vi "PH_Beckhoff_StepMot.calc Activity.vi"(1 "Endswitch?":bool, 2 "Moving":bool, 3 "ADS Error in":i32, 4 "Status":T1) -> (0 "Axis Activity":T4)   [LabVIEW 2014, in "PH_Beckhoff_StepMot.lvlib"]
uses:
  PH_Beckhoff_StepMot.lvlib
  PH_Stepmotor_BaseClass/PH_Stepmotor_BaseClass.Axis Activity.ctl
  non_GPL/instr.lib/Beckhoff/Read and Write Data/Step Motor Klemmen/Beckhoff.Step Motor - Status.ctl
  non_GPL/instr.lib/Beckhoff/Read and Write Data/Step Motor Klemmen/Beckhoff.Step Motor - Status Byte.ctl
  non_GPL/instr.lib/Beckhoff/Read and Write Data/Step Motor Klemmen/Beckhoff.Step Motor - Status Word.ctl
  PH_Stepmotor_BaseClass/PH_Stepmotor_BaseClass.lvlib
  non_GPL/instr.lib/Beckhoff/Beckhoff - Driver np.lvlib
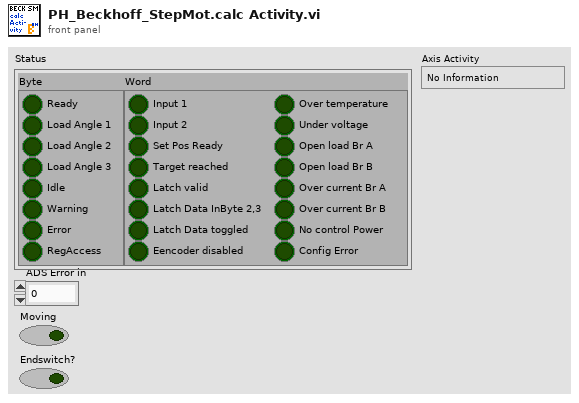
[diagram p1: front panel]
types:
  T1 = typedef "Beckhoff - Driver np.lvlib/Beckhoff.Step Motor - Status.ctl" = cluster{"Byte":T2, "Word":T3}
  T2 = typedef "Beckhoff - Driver np.lvlib/Beckhoff.Step Motor - Status Byte.ctl" = cluster{"Ready":bool, "Load Angle 1":bool, "Load Angle 2":bool, "Load Angle 3":bool, "Idle":bool, "Warning":bool, "Error":bool, "RegAccess":bool}
  T3 = typedef "Beckhoff - Driver np.lvlib/Beckhoff.Step Motor - Status Word.ctl" = cluster{"Input 1":bool, "Input 2":bool, "Set Pos Ready":bool, "Target reached":bool, "Latch valid":bool, "Latch Data InByte 2,3":bool, "Latch Data toggled":bool, "Eencoder disabled":bool, "Over temperature":bool, "Under voltage":bool, "Open load Br A":bool, "Open load Br B":bool, "Over current Br A":bool, "Over current Br B":bool, "No control Power":bool, "Config Error":bool}
  T4 = typedef "PH_Stepmotor_BaseClass.lvlib/PH_Stepmotor_BaseClass.Axis Activity.ctl" = enum16{"No Information", "stopped", "running", "Failure", "Alarm", "stopped at backward ES", "stopped at foreward ES"}
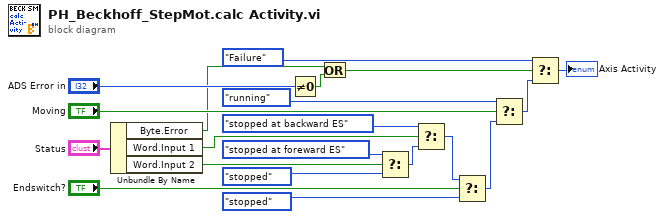
[diagram p0: block diagram]
diagram:
  n1 = Unbundle By Name("Status") -> ("Byte.Error"=w3:bool, "Word.Input 1"=w2:bool, "Word.Input 2"=w1:bool)
  n2 = Not Equal To 0?(x="ADS Error in") -> (x != 0?=w8:bool)
  n3 = Or(x=w3, y=w8) -> (x .or. y?=w6:bool)
  n4 = Select(t=PH_Stepmotor_BaseClass.Axis_Activity."stopped at foreward ES" ("Axis Activity"), s=w1, f=PH_Stepmotor_BaseClass.Axis_Activity."stopped") -> (s? t:f=w18:T4)
  n5 = Select(t=PH_Stepmotor_BaseClass.Axis_Activity."stopped at backward ES" ("Axis Activity"), s=w2, f=w18) -> (s? t:f=w17:T4)
  n6 = Select(t=w17, s="Endswitch?", f=PH_Stepmotor_BaseClass.Axis_Activity."stopped" ("Axis Activity")) -> (s? t:f=w15:T4)
  n7 = Select(t=PH_Stepmotor_BaseClass.Axis_Activity."running" ("Axis Activity"), s="Moving", f=w15) -> (s? t:f=w11:T4)
  n8 = Select(t=PH_Stepmotor_BaseClass.Axis_Activity."Failure" ("Axis Activity"), s=w6, f=w11) -> (s? t:f=→"Axis Activity":T4)
